vi "Save_Time_Traces.vi"() -> (5 "Plug in titles":string[](array[string]), 7 "Plug in values":string[](array[string]))   [LabVIEW 2010]
uses:
  Controls/Instrument_Array.ctl
  Globals/Meas_global.vi
panel:
  in  "No of desired samples/ch":i32
  in  "Down Sample":i32=1
  in  "File Extension":string=".xls"
  in  "Time Series":enum16{"Milliseconds", "Seconds"}(ring)
  in  "Full Header Info?":bool
  in  "Put each block into separate file":bool
  in  "Leave space between blocks?":bool
  in  "Precision":i16=2
  in  "Data to save":i32[](array[ring])=[1] items=["RV (C)", "Save Nothing"]
  in  "Separation Character":string="\t"
  # "Run this VI to update the channel names"
  # "You Must have selected the \"Save Data\" option on the \nMeasurement Program for this vi to save time traces"
  # "0 means disabled"
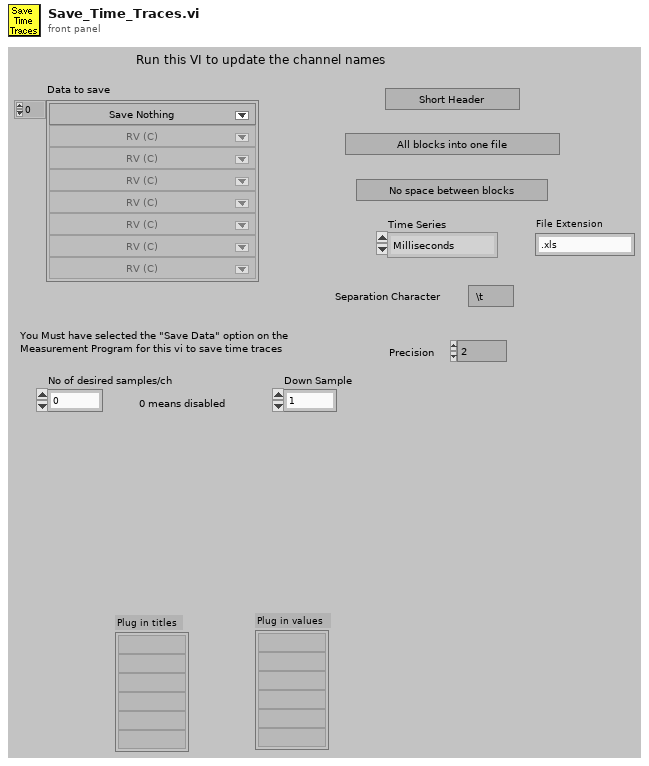
[diagram p1: front panel]
types:
  T1 = typedef "Analysis_info_cluster.ctl" = cluster{"Colour":u32, "Inst type":T2, "Inst name":string, "Symbol":string, "Code name":string, "Extra Info":string, "Inst Array":T3, "Index":i32, "Voltage Index":i32, "Extra Titles":string[], "Extra Values":string[]}
  T2 = typedef "Inst_type.ctl" = enum16{"Propeller anemometer", "Raw voltage", "Pressure Transducer", "Pitot-static tube", "Preston tube", "Hot wire", "Cross wire 1", "Cross wire 2", "Generic Linear", "Generic Polynomial", "Generic BackPoly", "Fast FID", "Thermocouple", "Cold wire", "Pulsed Wire", "LDA Vel", "LDA Tran time", "LDA Arr time"}
  T3 = typedef "Instrument_Array.ctl" = enum16{"PWA", "LDA", "Analogue"}
  T4 = enum16{"Save no data", "Save data in new files", "Save data in existing files"}
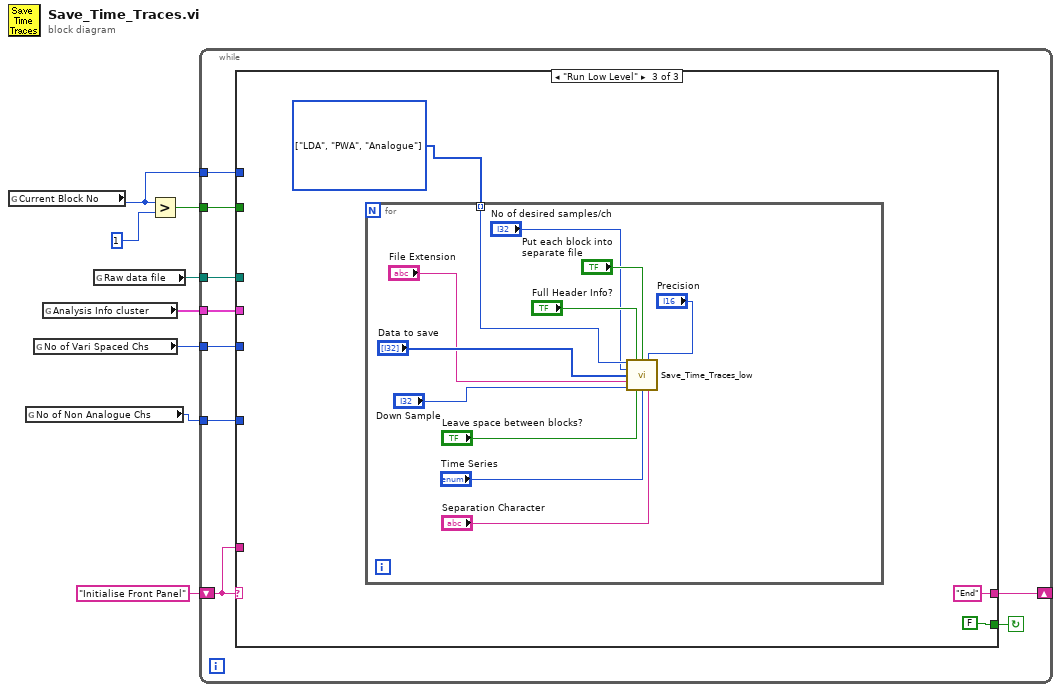
[diagram p0: block diagram]
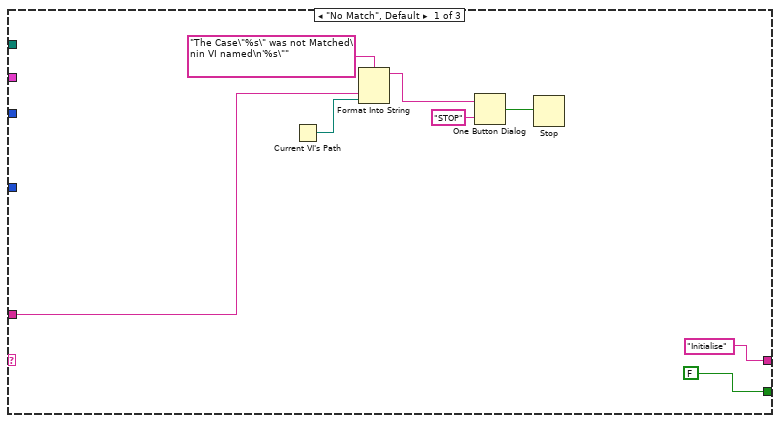
[diagram p2: hidden frame]
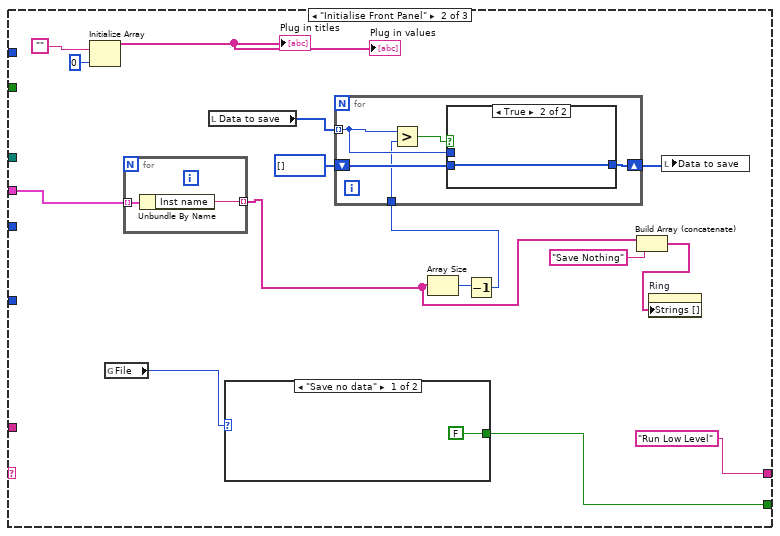
[diagram p3: hidden frame]
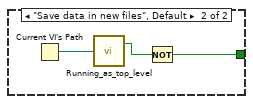
[diagram p4: hidden frame]
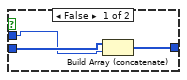
[diagram p5: hidden frame]
diagram:
  n1 = global read "Meas_global.vi" "Current Block No"() -> (w4:i32)
  n2 = global read "Meas_global.vi" "No of Non Analogue Chs"() -> (w1:i32)
  n3 = global read "Meas_global.vi" "No of Vari Spaced Chs"() -> (w2:i32)
  n4 = global read "Meas_global.vi" "Analysis Info cluster"() -> (w3:T1[])
  n5 = global read "Meas_global.vi" "Raw data file"() -> (w7:path)
  n6 = Greater?(x=w4, y=1) -> (0:w5:bool)
  n7 = while {
    shift-left: "Initialise Front Panel" -> [w15]
    shift-right: [w16] -> _
    tunnel: w7 -> [w14]
    tunnel: w5 -> [w13]
    tunnel: w4 -> [w12]
    tunnel: w3 -> [w11]
    tunnel: w2 -> [w10]
    tunnel: w1 -> [w9]
    stop <- w17 continue-if-true
    n8 = case shown="\"Run Low Level\"" w15 {
      tunnel: [FALSE w26 FALSE] -> w17
      tunnel: ["Initialise" "Run Low Level" ("t") "End" ("t")] -> w16
      tunnel: w15 -> [w20 _ _]
      tunnel: w14 -> [_ _ _]
      tunnel: w13 -> [_ _ _]
      tunnel: w12 -> [_ _ _]
      tunnel: w11 -> [_ w37 _]
      tunnel: w10 -> [_ _ _]
      tunnel: w9 -> [_ _ _]
      frame "No Match", Default {
        n9 = Current VI's Path() -> (path=w19:path)
        n10 = Format Into String(format string="The Case\"%s\" was not Matched\nin VI named\n'%s\"" ("Format String"), w20, w19) -> (resulting string=w23:string)  [unwired: 2 in, 1 out]
        n11 = One Button Dialog(message=w23, button name ("OK")="STOP") -> (true=w21:bool)
        n12 = Stop(stop? (T)=w21) -> ()
      }
      frame "Initialise Front Panel" {
        n13 = Initialize Array("", 0) -> (→"Plug in values" →"Plug in titles":string[])
        n14 = global read "Meas_global.vi" "File"() -> (w27:T4)
        n15 = for {
          tunnel: w37 -> [w55] mode=indexing
          tunnel: [w54] -> w29 mode=indexing
          n16 = Unbundle By Name(w55) -> ("Inst name"=w54:string)
        }
        n17 = local read "Data to save"() -> (w36:i32[])
        n18 = case shown="\"Save no data\"" w27 {
          tunnel: [FALSE w42] -> w26
          frame "Save no data" {
          }
          frame "Save data in new files", Default {
            n19 = Current VI's Path() -> (path=w43:path)
            n20 = call "Running_as_top_level.vi"("Vi path name"=w43) -> ("Top Level"=w44:bool)  [unwired: 1 out]
            n21 = Not(x=w44) -> (.not. x?=w42:bool)
          }
        }
        n22 = Array Size(array=w29) -> (size(s)=w31:i32)
        n23 = Decrement(x=w31) -> (x-1=w30:i32)
        n24 = for {
          tunnel: w36 -> [w46] mode=indexing
          shift-right: [w47] -> w34
          shift-left: i32[] [] -> [w48]
          tunnel: w30 -> [w45]
          n25 = Greater?(x=w46, y=w45) -> (0:w49:bool)
          n26 = case shown="True" w49 {
            tunnel: w48 -> [w52 w53]
            tunnel: [w51 w53] -> w47
            tunnel: w46 -> [w50 _]
            frame False {
              n27 = Build Array (concatenate)(w52, w50) -> (w51:i32[])
            }
            frame True {
            }
          }
        }
        n28 = Build Array (concatenate)(w29, "Save Nothing") -> (w32:string[])
        n29 = property on="Ring" class="Ring (strict)"("Strings []"=w32) -> ()  [unwired: 2 in, 2 out]
        n30 = local write "Data to save"(w34) -> ()
      }
      frame "Run Low Level" {
        w57 = T3[] [enum."LDA", enum."PWA", enum."Analogue"] items=["PWA", "LDA", "Analogue"]
        n31 = for {
          tunnel: w57 -> [w62] mode=indexing
          n32 = call "Save_Time_Traces_low.vi"("Data Type"=w62, "Full Header Info?"="Full Header Info?", "Put each block into separate file"="Put each block into separate file", "Precision"="Precision", "No of desired samples/ch"="No of desired samples/ch", "Data to save"="Data to save", "File Extension"="File Extension", "Down Sample"="Down Sample", "Leave space between blocks?"="Leave space between blocks?", "Time Series"="Time Series", "Separation Character"="Separation Character") -> ()  [unwired: 5 out]
        }
      }
    }
  }
